vi "Teleop.vi"(10 "Match Info":T1={"Autonomous Elapsed Seconds"=0.0, "TeleOp Elapsed Seconds"=0.0, "Disabled Elapsed Seconds"=0.0, "Visited Autonomous"=FALSE, "Visited TeleOp"=FALSE, "Visited Disabled"=FALSE, "Autonomous Settings"={"Autonomous Style"=enum."Independent", "VI Refnum"=refnum}}, 11 "Call Context":T2) -> ()   [LabVIEW 2016]
doc: "This VI is called for each TeleOp packet received from the DS where the robot is not disabled. It is often used to read from the joysticks and update I/O or to update setpoints for timed control loops. It should complete and return within 20 milliseconds or it may miss DS packets."
uses:
  <vilib>/Rock Robotics/WPI/DriverStation/WPI_DriverStationDerivedRobotMode.ctl
  <vilib>/Rock Robotics/WPI/DriverStation/WPI_DriverStationMatch Info.ctl
  <vilib>/Rock Robotics/Network Tables/NT Read Boolean.vi
  Robot Global Data.vi
  <vilib>/Rock Robotics/Network Tables/NT Read Number.vi
  <vilib>/Rock Robotics/Network Tables/NT Write Boolean Array.vi
  <vilib>/Rock Robotics/Network Tables/NT Write Numeric Array.vi
panel:
  out "Sample Slider 0":dbl(slide) scale=0.0..5.0
  out "Sample Boolean 1":bool
  out "Sample Boolean 0":bool
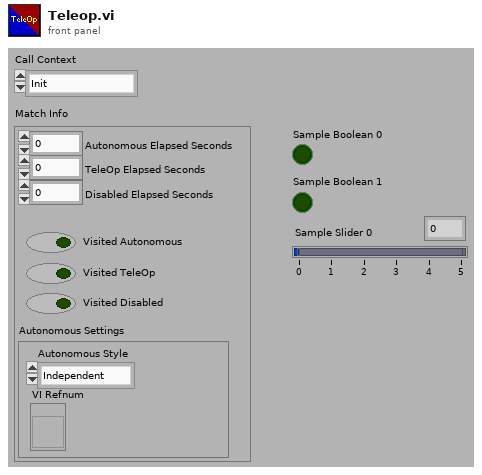
[diagram p1: front panel]
types:
  T1 = typedef "WPI_DriverStationMatch Info.ctl" = cluster{"Autonomous Elapsed Seconds":dbl, "TeleOp Elapsed Seconds":dbl, "Disabled Elapsed Seconds":dbl, "Visited Autonomous":bool, "Visited TeleOp":bool, "Visited Disabled":bool, "Autonomous Settings":cluster{"Autonomous Style":enum16{"Iterative", "Independent"}, "VI Refnum":refnum<vi>}}
  T2 = typedef "WPI_DriverStationDerivedRobotMode.ctl" = enum16{"Init", "Execute", "Stop"}
  T3 = typedef "WPI_JoystickDevRef.ctl" = cluster{"Device":T4}
  T4 = typedef "WPI_JoystickDeviceEnum.ctl" = enum16{"USB 0", "USB 1", "USB 2", "USB 3", "USB 4", "USB 5"}
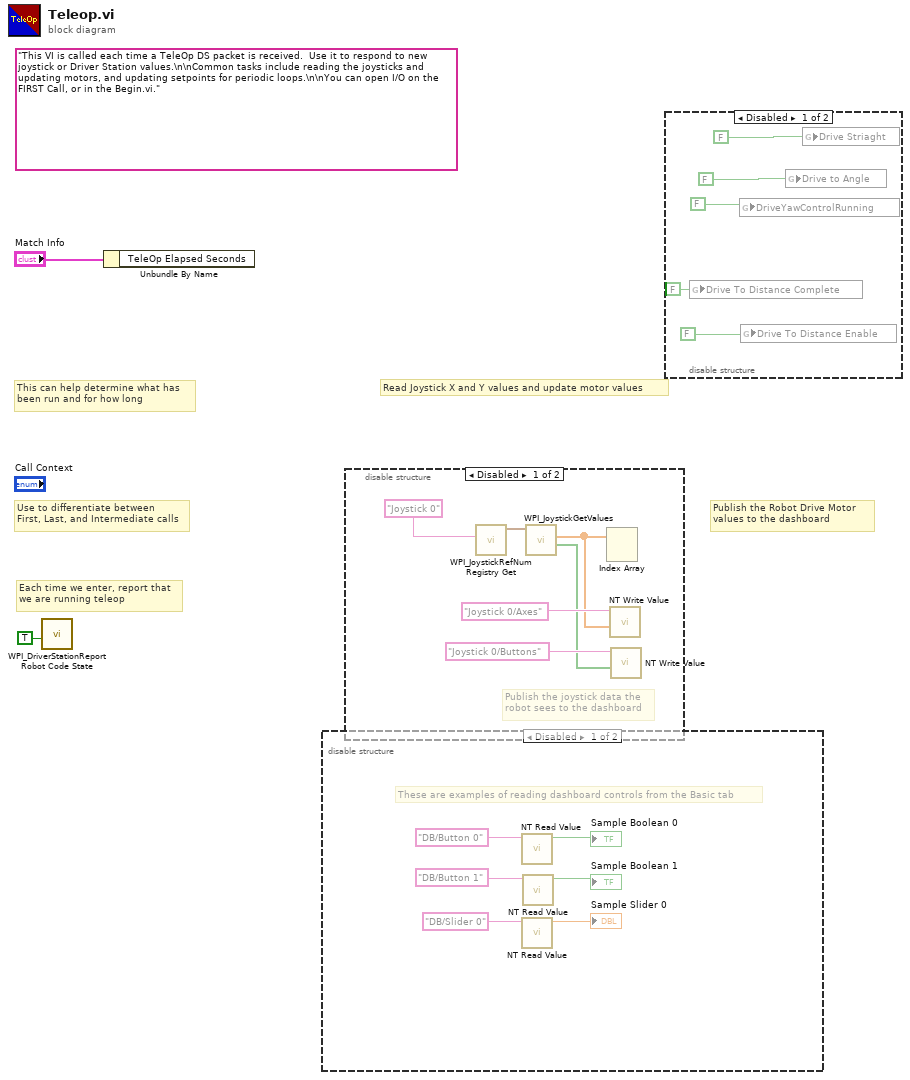
[diagram p0: block diagram]
diagram:
  (unwired) "This VI is called each time a TeleOp DS packet is received.  Use it to respond to new joystick or Driver Station values.\n\nCommon tasks include reading the joysticks and updating motors, and updating setpoints for periodic loops.\n\nYou can open I/O on the FIRST Call, or in the Begin.vi."
  # "Publish the Robot Drive Motor\nvalues to the dashboard"
  # "Each time we enter, report that\nwe are running teleop"
  # "Use to differentiate between\nFirst, Last, and Intermediate calls"
  # "This can help determine what has\nbeen run and for how long"
  # "Read Joystick X and Y values and update motor values"
  n1 = call <vilib>:"WPI_DriverStationReport Robot Code State.vi"("TeleOp"=TRUE ("Autonomous")) -> ()  [unwired: 10 in, 1 out]
  n2 = Unbundle By Name("Match Info") -> ()  [unwired: 1 out]
  n3 = disable-structure shown="Disabled" {
    frame Disabled {
      # "These are examples of reading dashboard controls from the Basic tab"
      n4 = call-poly <vilib>:"NT Read Value.vi"("Name"="DB/Button 0" ("refnum name")) -> ("Boolean"=→"Sample Boolean 0":bool)  [unwired: 9 in, 1 out]
      n5 = call-poly <vilib>:"NT Read Value.vi"("Name"="DB/Slider 0" ("refnum name")) -> ("Numeric"=→"Sample Slider 0":dbl)  [unwired: 9 in, 1 out]
      n6 = call-poly <vilib>:"NT Read Value.vi"("Name"="DB/Button 1" ("refnum name")) -> ("Boolean"=→"Sample Boolean 1":bool)  [unwired: 9 in, 1 out]
    }
    frame Enabled {
    }
  }
  n7 = disable-structure shown="Disabled" {
    frame Disabled {
      # "Publish the joystick data the\nrobot sees to the dashboard"
      n8 = call <vilib>:"WPI_JoystickRefNum Registry Get.vi"("refnum name"="Joystick 0") -> ("JoystickDevRef"=w13:T3)  [unwired: 1 in, 9 out]
      n9 = call <vilib>:"WPI_JoystickGetValues.vi"("JoystickDevRef"=w13) -> ("Buttons"=w9:bool[], "Axes"=w10:dbl[])  [unwired: 6 in, 3 out]
      n10 = Index Array(array=w10) -> ()  [unwired: 2 in, 2 out]
      n11 = call-poly <vilib>:"NT Write Value.vi"("Numeric Array"=w10, "Name"="Joystick 0/Axes") -> ()  [unwired: 9 in, 1 out]
      n12 = call-poly <vilib>:"NT Write Value.vi"("Boolean Array"=w9, "Name"="Joystick 0/Buttons") -> ()  [unwired: 9 in, 1 out]
    }
    frame Enabled {
    }
  }
  n13 = disable-structure shown="Disabled" {
    frame Disabled {
      n14 = global write "Robot Global Data.vi" "Drive To Distance Complete"(FALSE ("Drive To Distance Complete")) -> ()
      n15 = global write "Robot Global Data.vi" "DriveYawControlRunning"(FALSE ("DriveYawControlRunning")) -> ()
      n16 = global write "Robot Global Data.vi" "Drive To Distance Enable"(FALSE ("Drive To Distance Enable")) -> ()
      n17 = global write "Robot Global Data.vi" "Drive to Angle"(FALSE ("Drive To Distance Enable")) -> ()
      n18 = global write "Robot Global Data.vi" "Drive Striaght"(FALSE ("Drive To Distance Enable")) -> ()
    }
    frame Enabled {
    }
  }
